vi "New fruit.vi"(8 "error in (no error)":errorcluster, 10 "Color":u32(colorbox), 11 "Fruit in":refnum<class "Fruit.lvclass">) -> (0 "error out":errorcluster, 3 "Fruit out":refnum<class "Fruit.lvclass">)   [LabVIEW 2021, in "Fruit.lvclass"]
uses:
  Fruit.lvclass
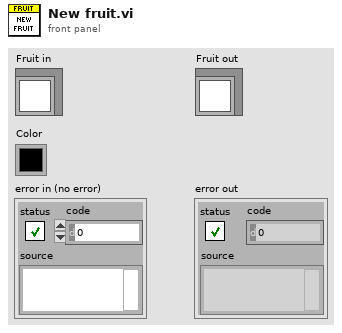
[diagram p1: front panel]
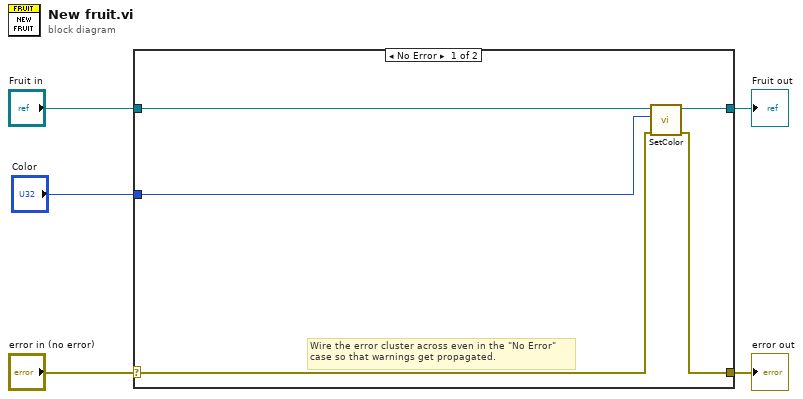
[diagram p0: block diagram]
diagram:
  n1 = case shown="No Error" "error in (no error)" {
    selector: "error in (no error)" -> [w7 w12]
    tunnel: [w6 w12] -> w4
    tunnel: [w9 w11] -> w2
    tunnel: "Fruit in" -> [w10 w11]
    tunnel: "Color" -> [w8 _]
    frame No Error {
      # "Wire the error cluster across even in the \"No Error\"\ncase so that warnings get propagated."
      n2 = call-dynamic "SetColor.vi"("error in (no error)"=w7, "Color"=w8, "SnakeGame in"=w10) -> ("error out"=w6:errorcluster, "SnakeGame out"=w9:refnum<class "Fruit.lvclass">)  [unwired: 7 in]
    }
    frame Error {
    }
  }
  "error out" <- w4
  "Fruit out" <- w2
